vi "Solve1.vi"(8 "Error In":errorcluster, 11 "object in":refnum<class "2024_6.lvclass">) -> (0 "Error Out":errorcluster, 2 "Result":u64, 3 "object out":refnum<class "2024_6.lvclass">)   [LabVIEW 2023, in "2024_6.lvclass"]
uses:
  2024_6.lvclass
  2024_6.lvclass/2024_6.ctl
  <vilib>/Utility/miscctls.llb/LVMapReplaceAction.ctl
panel:
  out "Enum":enum16{"Up", "Right", "Down", "Left"}(ring)
  out "map":u32[][](array[colorbox])
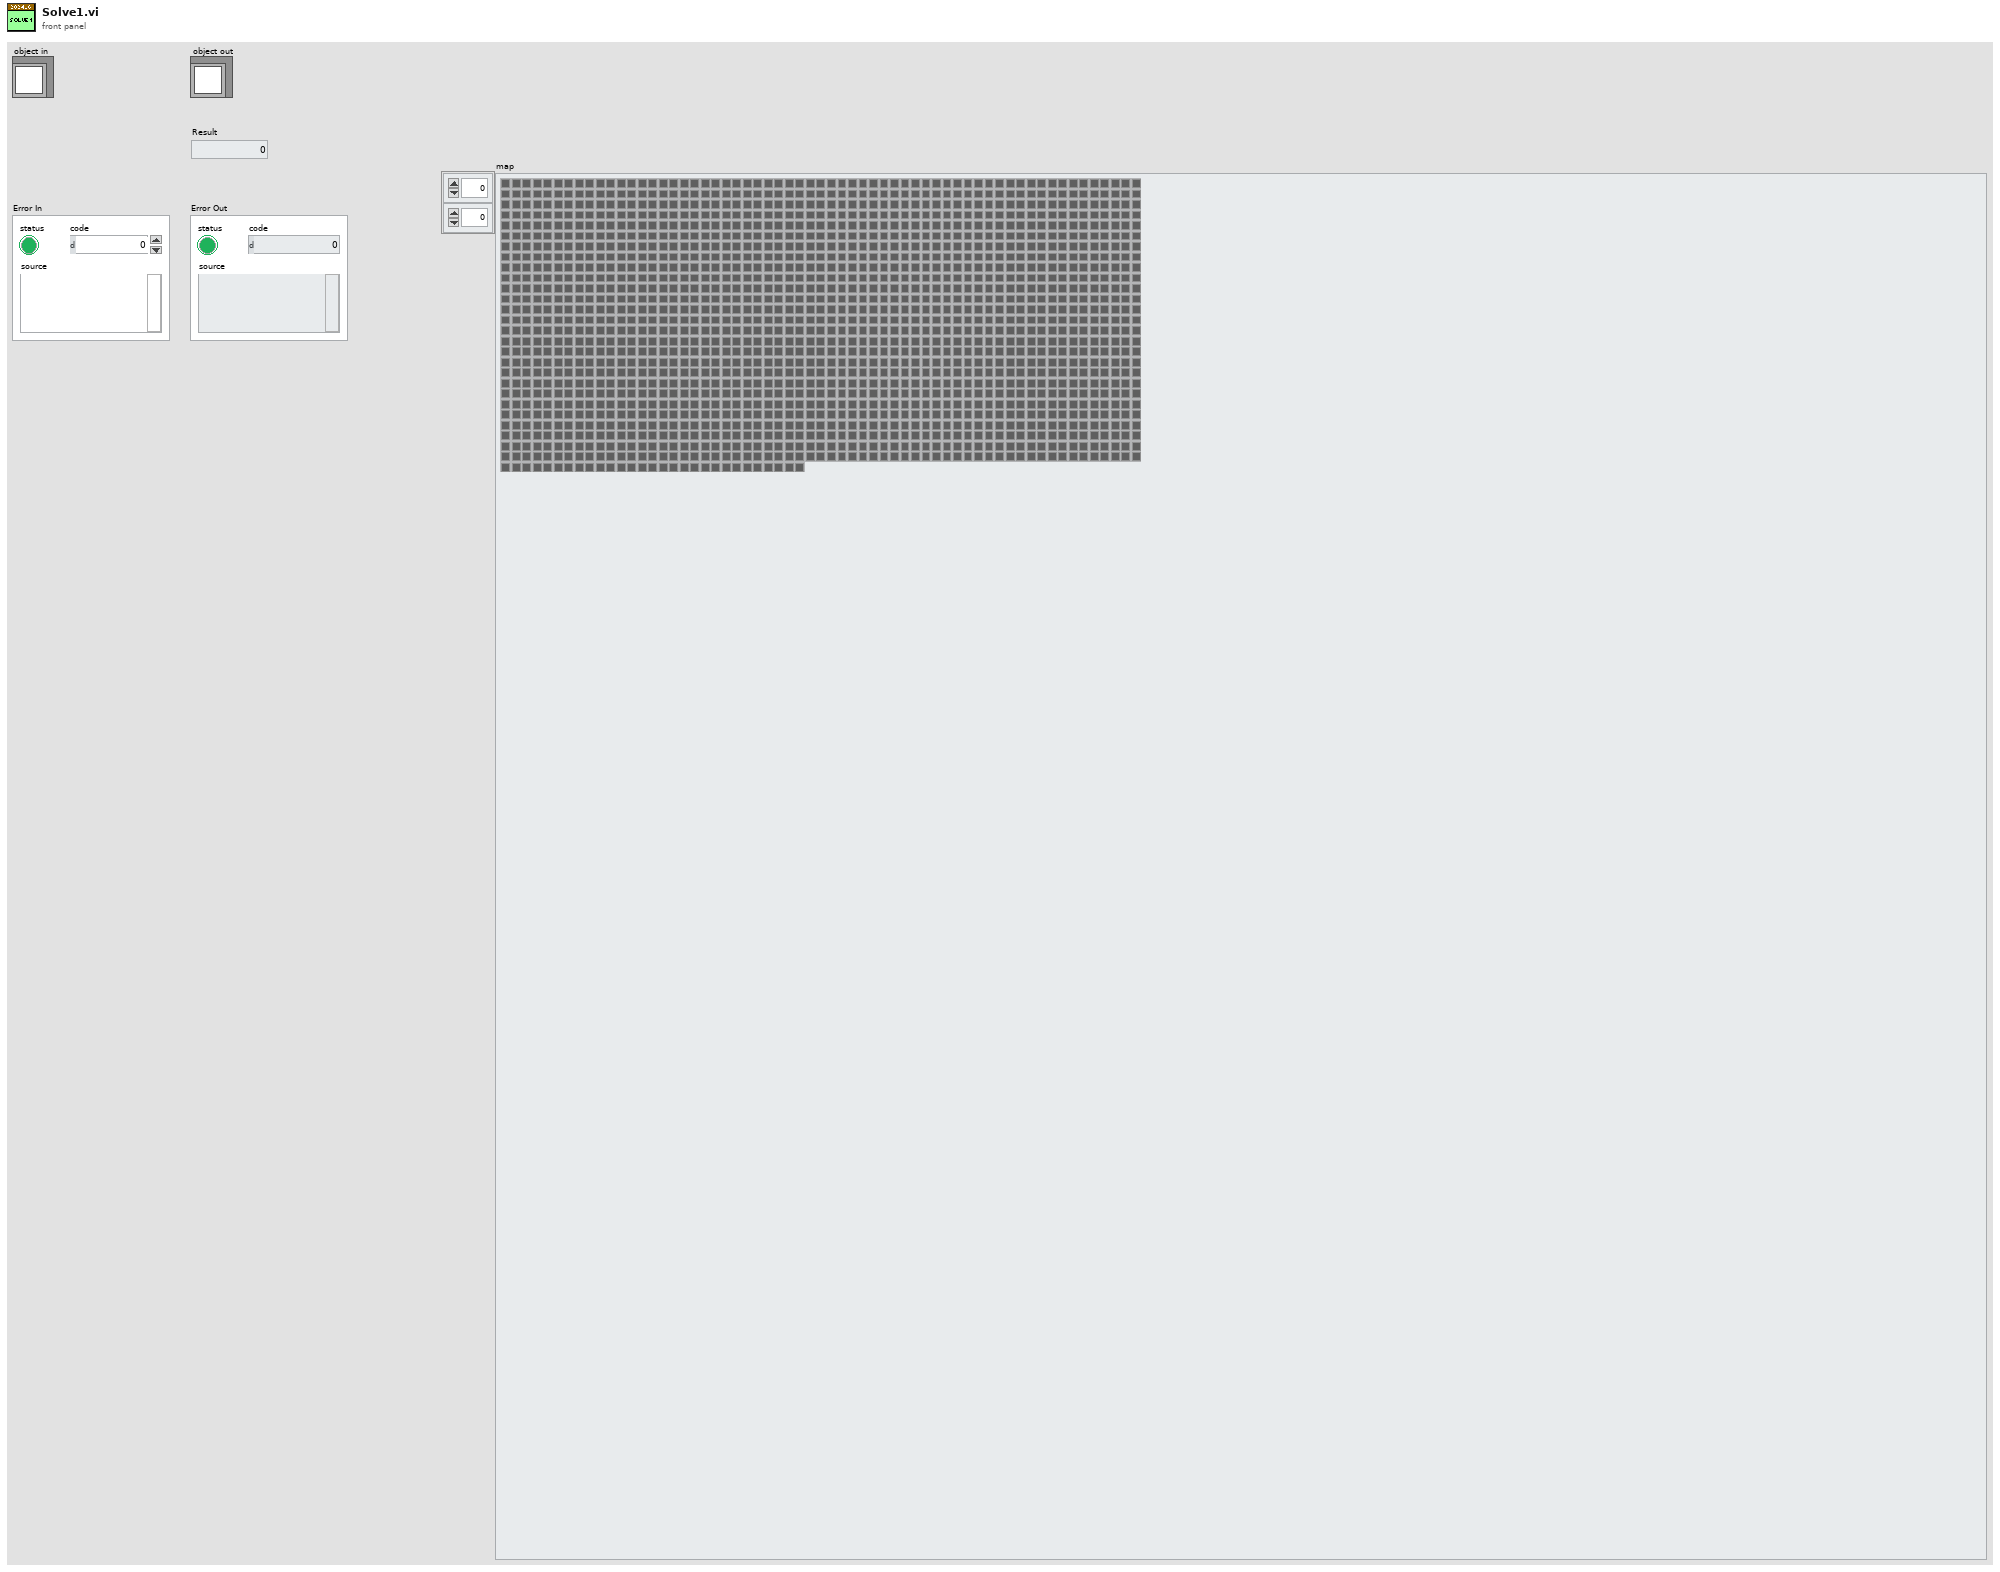
[diagram p1: front panel]
types:
  T1 = typedef "LVMapReplaceAction.ctl" = enum32{"Modify Entry only if found", "Add or Modify Entry", "Delete Entry"}
  T2 = map{cluster{"X":i32, "Y":i32}, set{enum16{"Up", "Right", "Down", "Left"}}}
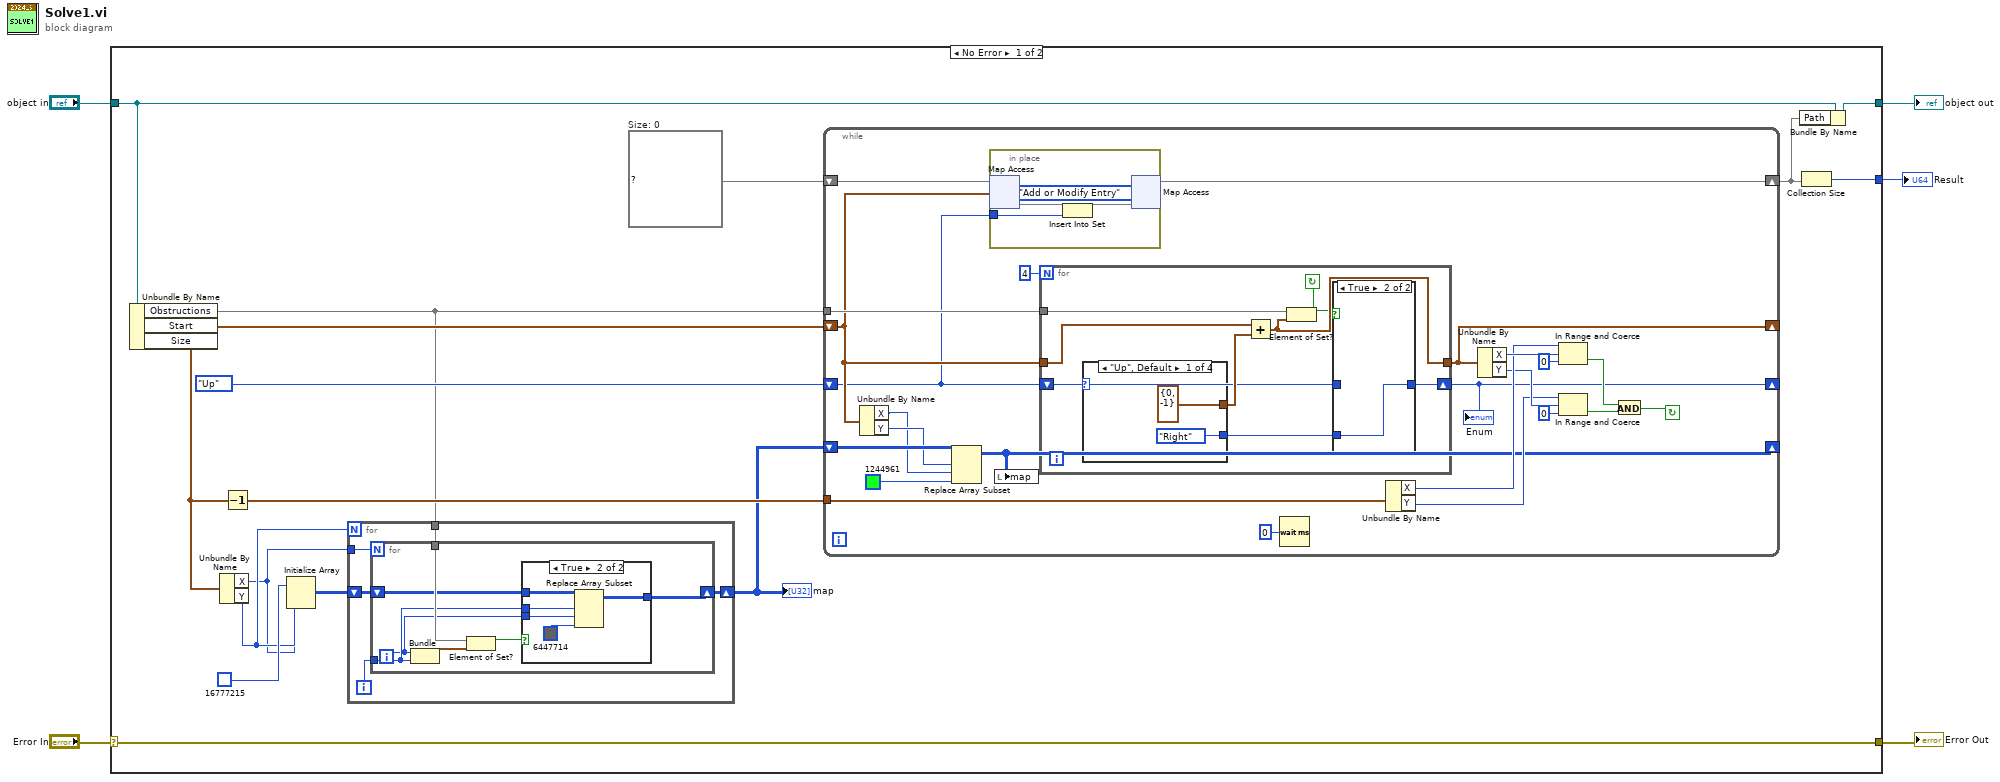
[diagram p0: block diagram]
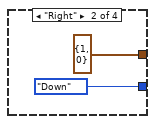
[diagram p4: hidden frame]
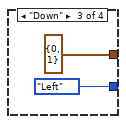
[diagram p5: hidden frame]
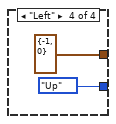
[diagram p6: hidden frame]
diagram:
  n1 = case shown="No Error" "Error In" {
    selector: "Error In" -> [w21 w87]
    tunnel: [w21 w87] -> w4
    tunnel: [w8 w86] -> w2
    tunnel: "object in" -> [w20 w86]
    tunnel: [w16 _] -> w1
    frame No Error {
      w7 = T2 {}  # Size: 0
      n2 = Unbundle By Name(w20) -> ("Obstructions"=w12:set{cluster{"X":i32, "Y":i32}}, "Start"=w19:cluster{"X":i32, "Y":i32}, "Size"=w15:cluster{"X":i32, "Y":i32})
      n3 = Unbundle By Name(w15) -> ("X"=w10:i32, "Y"=w11:i32)
      n4 = Decrement(x=w15) -> (x-1=w17:cluster{"X":i32, "Y":i32})
      n5 = Initialize Array(u32 16777215, w11, w10) -> (w13:u32[][])
      n6 = for {
        N: w11 -> [_]
        tunnel: w12 -> [w24]
        shift-right: [w22] -> w9
        shift-left: w13 -> [w26]
        tunnel: w10 -> [w23]
        i -> [w25]
        n7 = for {
          N: w23 -> [_]
          tunnel: w25 -> [w29]
          tunnel: w24 -> [w33]
          shift-right: [w27] -> w22
          shift-left: w26 -> [w30]
          i -> [w28]
          n8 = Bundle(w28, w29) -> (w32:cluster{i32, i32})  [unwired: 1 in]
          n9 = Element of Set?(10:w32, 11:w33) -> (3:w31:bool)
          n10 = case shown="True" w31 {
            tunnel: w30 -> [w34 w39]
            tunnel: w29 -> [_ w38]
            tunnel: w28 -> [_ w37]
            tunnel: [w34 w35] -> w27
            frame False {
            }
            frame True {
              n11 = Replace Array Subset(array=w39, new element=u32 6447714, index (row)=w38, index (col)=w37) -> (w35:u32[][])
            }
          }
        }
      }
      "map" <- w9
      n12 = while {
        shift-right: [w51] -> _
        shift-left: w19 -> [w41]
        shift-right: [w50] -> _
        shift-left: enum16{"Up", "Right", "Down", "Left"}."Up" -> [w40]
        shift-right: [w42] -> w6
        shift-left: w7 -> [w43]
        tunnel: w17 -> [w61]
        tunnel: w12 -> [w56]
        shift-right: [w45] -> _
        shift-left: w9 -> [w49]
        stop <- w52 continue-if-true
        n13 = Unbundle By Name(w41) -> ("X"=w47:i32, "Y"=w48:i32)
        n14 = Replace Array Subset(array=w49, new element=u32 1244961, index (row)=w48, index (col)=w47) -> (w45:u32[][])
        n15 = in-place {
          in-place-border: w40 -> [w66]
          n16 = in-place-map #1(w43, w41) -> (w67:set{enum16{"Up", "Right", "Down", "Left"}})  [unwired: 1 in, 1 out]
          n17 = Insert Into Set(10:w66, 11:w67) -> (3:w65:set{enum16{"Up", "Right", "Down", "Left"}})  [unwired: 1 out]
          n18 = in-place-map #1(w65, LVMapReplaceAction."Add or Modify Entry" ("action")) -> (w42:T2)  [unwired: 2 out]
        }
        n19 = local write "map"(w45) -> ()
        n20 = for {
          N: 4 -> [_]
          tunnel: w56 -> [w73]
          shift-right: [w69] -> w50
          shift-left: w40 -> [w70]
          tunnel: w41 -> [w75]
          tunnel: [w72] -> w51
          stop <- w71 continue-if-true
          n21 = case shown="\"Up\", Default" w70 {
            tunnel: [cluster{"X":i32, "Y":i32} {"X"=0, "Y"=-1} ("y") cluster{"X":i32, "Y":i32} {"X"=1, "Y"=0} ("y") cluster{"X":i32, "Y":i32} {"X"=0, "Y"=1} ("y") cluster{"X":i32, "Y":i32} {"X"=-1, "Y"=0} ("y")] -> w74
            tunnel: [enum16{"Up", "Right", "Down", "Left"}."Right" enum16{"Up", "Right", "Down", "Left"}."Down" enum16{"Up", "Right", "Down", "Left"}."Left" enum16{"Up", "Right", "Down", "Left"}."Up"] -> w68
            frame "Up", Default {
            }
            frame "Right" {
            }
            frame "Down" {
            }
            frame "Left" {
            }
          }
          n22 = Add(x=w75, y=w74) -> (x+y=w72:cluster{"X":i32, "Y":i32})
          n23 = Element of Set?(10:w72, 11:w73) -> (3:w71:bool)
          n24 = case shown="True" w71 {
            tunnel: w70 -> [w76 _]
            tunnel: [w76 w77] -> w69
            tunnel: w68 -> [_ w77]
            frame False {
            }
            frame True {
            }
          }
        }
        "Enum" <- w50
        n25 = Wait (ms)(milliseconds to wait=u32 0) -> ()  [unwired: 1 out]
        n26 = Unbundle By Name(w61) -> ("X"=w60:i32, "Y"=w57:i32)
        n27 = Unbundle By Name(w51) -> ("X"=w63:i32, "Y"=w58:i32)
        n28 = In Range and Coerce(upper limit=w60, x=w63, lower limit=0) -> (In Range?=w53:bool)  [unwired: 1 out]
        n29 = In Range and Coerce(upper limit=w57, x=w58, lower limit=0) -> (In Range?=w54:bool)  [unwired: 1 out]
        n30 = And(x=w53, y=w54) -> (x .and. y?=w52:bool)
      }
      n31 = Bundle By Name(cluster=w20, "Path"=w6) -> (w8:refnum<class "2024_6.lvclass">)
      n32 = Collection Size(1:w6) -> (0:w16:i32)
    }
    frame Error {
    }
  }
  "Error Out" <- w4
  "object out" <- w2
  "Result" <- w1
